vi "HTS_READY.vi"(8 "Error IN":errorcluster, 11 "VISA resource IN":refnum<visa-resource-name>="HTS") -> (0 "Error OUT":errorcluster, 1 "RESPONSE":string[](array[string])=["SYSTEM STATUS: ", "0x0", "2 PUMPS", "PUMP_1 STATUS: ", "0x60", "PUMP_2 STATUS: ", "0x60", "AXIS X STATUS: ", "0x9", "AXIS Y STATUS: ", "0x9", "AXIS P STATUS: ", "0x9", "AXIS Z STATUS: ", "0x9", "NO ERROR, READY", ">"], 2 "READY?":bool=TRUE, 3 "VISA resource OUT":refnum<visa-resource-name>="HTS")   [LabVIEW 2013]
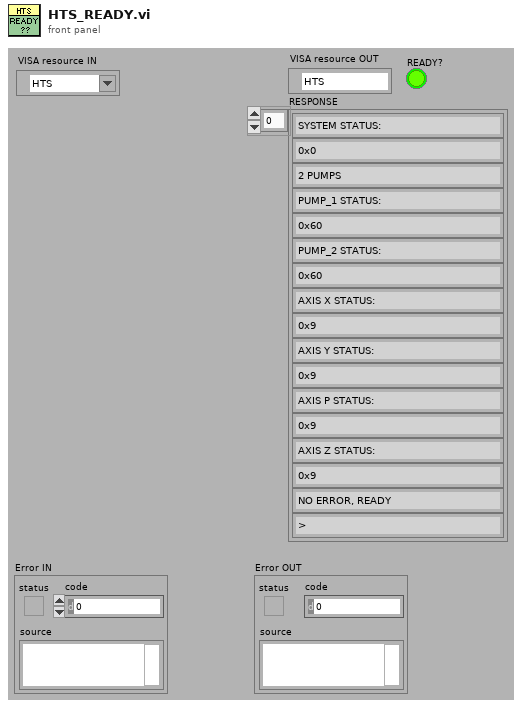
[diagram p1: front panel]
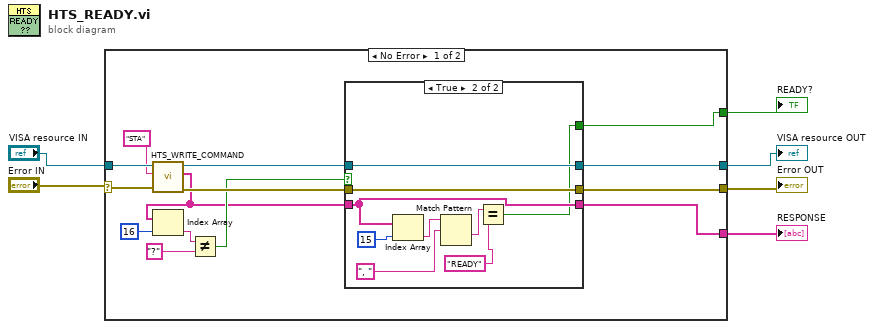
[diagram p0: block diagram]
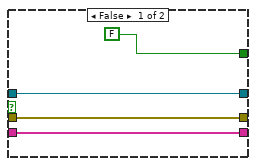
[diagram p2: hidden frame]
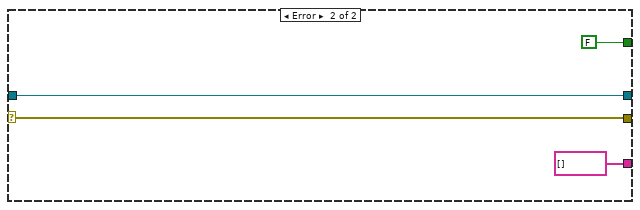
[diagram p3: hidden frame]
diagram:
  n1 = case shown="No Error" "Error IN" {
    selector: "Error IN" -> [w20 w37]
    tunnel: [w10 w37] -> w5
    tunnel: "VISA resource IN" -> [w19 w36]
    tunnel: [w14 w36] -> w3
    tunnel: [w7 FALSE] -> w2
    tunnel: [w8 string[] [] ("RESPONSE")] -> w1
    frame No Error {
      n2 = call "HTS_WRITE_COMMAND.vi"("Error IN"=w20, "Command"="STA", "HTS PORT IN"=w19) -> ("Error OUT"=w16:errorcluster, "RESPONSE"=w9:string[], "HTS PORT OUT"=w15:refnum<visa-resource-name>)  [unwired: 6 out]
      n3 = Index Array(array=w9, index=16) -> (element=w13:string)
      n4 = Not Equal?(x=w13, y="?") -> (x != y?=w11:bool)
      n5 = case shown="True" w11 {
        tunnel: w16 -> [w23 w28]
        tunnel: w15 -> [w24 w29]
        tunnel: [w24 w29] -> w14
        tunnel: w9 -> [w22 w27]
        tunnel: [w23 w28] -> w10
        tunnel: [w22 w27] -> w8
        tunnel: [FALSE w26] -> w7
        frame False {
        }
        frame True {
          n6 = Index Array(array=w27, index=15) -> (element=w32:string)
          n7 = Match Pattern(string=w32, regular expression=", ") -> (after substring=w25:string)  [unwired: 4 out]
          n8 = Equal?(x=w25, y="READY" ("x")) -> (x = y?=w26:bool)
        }
      }
    }
    frame Error {
    }
  }
  "Error OUT" <- w5
  "VISA resource OUT" <- w3
  "READY?" <- w2
  "RESPONSE" <- w1
